vi "Translate.vi"   [LabVIEW 2011, in "PolarVector.lvclass"]
uses:
  PolarVector.lvclass
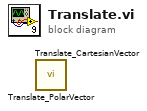
[diagram p0: block diagram]
diagram:
  n1 = call "Translate_PolarVector.vi"() -> ()  [unwired: 10 in, 2 out]
  n2 = call "Translate_CartesianVector.vi"() -> ()  [unwired: 10 in, 2 out]
